vi "PH_Calorimeter_USB.Calc Integral.vi"(1 "Time scale [s]":dbl[](array[numeric]) format="%.2f", 2 "T 1/E [s]":dbl=12.93 format="%.2f", 3 "Integration Time [s]":dbl=8.3 format="%.2f", 4 "Sample Rate [Hz]":dbl=10.0 format="%.2f", 5 "Data without Offset":sgl[](array[numeric]) format="%.2f") -> (17 "Integral value":dbl format="%.2f")   [LabVIEW 2014, in "PH_Calorimeter_USB.lvlib"]
doc: "This VI calculates the \"Integral value\". For this the following formula is used:\n\nMinimum of |\"time in\" - (\"T 1/E\" + \"integration time in\")| is the number of times a for loop is done. Within this the integral value is cal ulated in a funny way."
uses:
  PH_Calorimeter_USB.lvlib
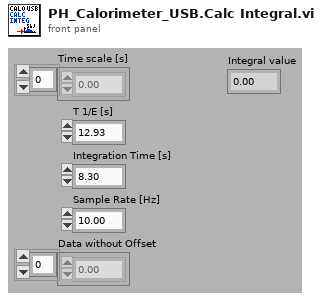
[diagram p1: front panel]
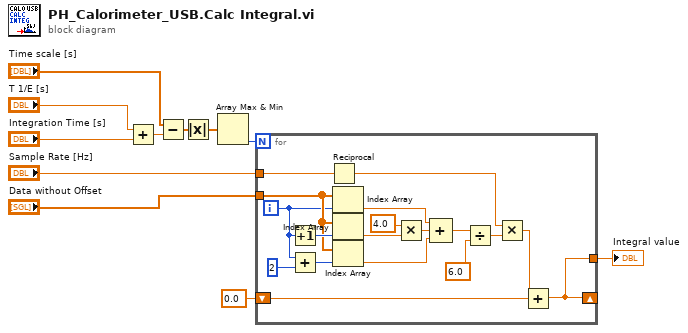
[diagram p0: block diagram]
diagram:
  n1 = Add(x="T 1/E [s]", y="Integration Time [s]") -> (x+y=w11:dbl)
  n2 = Subtract(x="Time scale [s]", y=w11) -> (x-y=w8:dbl[])
  n3 = Absolute Value(x=w8) -> (abs(x)=w7:dbl[])
  n4 = Array Max & Min(array=w7) -> (min index (indices)=w9:i32)  [unwired: 3 out]
  n5 = for {
    N: w9 -> [_]
    tunnel: "Data without Offset" -> [w24]
    shift-right: [w13] -> _
    shift-left: 0.0 -> [w18]
    tunnel: [w13] -> w3
    tunnel: "Sample Rate [Hz]" -> [w12]
    i -> [w14]
    n6 = Increment(x=w14) -> (x+1=w29:i32)
    n7 = Add(x=w14, y=2) -> (x+y=w28:i32)
    n8 = Reciprocal(x=w12) -> (1/x=w15:dbl)
    n9 = Index Array(array=w24, index=w14) -> (element=w22:sgl)
    n10 = Index Array(array=w24, index=w29) -> (element=w25:sgl)
    n11 = Index Array(array=w24, index=w28) -> (element=w21:sgl)
    n12 = Multiply(x=4.0, y=w25) -> (x*y=w23:dbl)
    n13 = Compound Arithmetic op=ADD(w22, w23, w21) -> (w20:dbl)
    n14 = Divide(x=w20, y=6.0) -> (x/y=w16:dbl)
    n15 = Multiply(x=w15, y=w16) -> (x*y=w17:dbl)
    n16 = Add(x=w17, y=w18) -> (x+y=w13:dbl)
  }
  "Integral value" <- w3
